vi "CODMn手动控制框.vi"(8 "Error in":errorcluster) -> ()   [LabVIEW 2016, in "斯坦道CODMn.lvlib"]
uses:
  <vilib>/Plasmionique/MB Master/MB Master.lvlib
panel:
  in  "氢氧化钠":bool
  in  "进样泵反转":bool
  in  "采水泵排":bool
  in  "采水泵进":bool
  in  "草酸钠":bool
  in  "高锰酸钾":bool
  in  "高锰酸钾滴定（10uL每滴）":bool
  in  "草酸钠泵排":bool
  in  "草酸钠泵进":bool
  in  "草酸钠泵复位":bool
  in  "高锰酸钾泵排":bool
  in  "高锰酸钾泵进":bool
  in  "高锰酸钾泵复位":bool
  in  "风扇":bool
  in  "排液":bool
  in  "搅拌":bool
  in  "加热":bool
  in  "硫酸":bool
  in  "加标回收样":bool
  in  "零点核查样":bool
  in  "标液":bool
  in  "纯水":bool
  in  "退出":bool
  in  "水样":bool
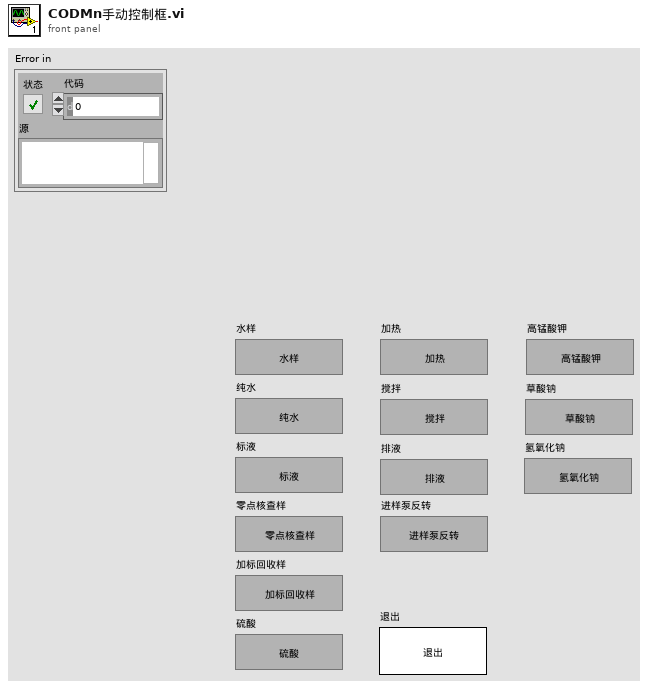
[diagram p1: front panel]
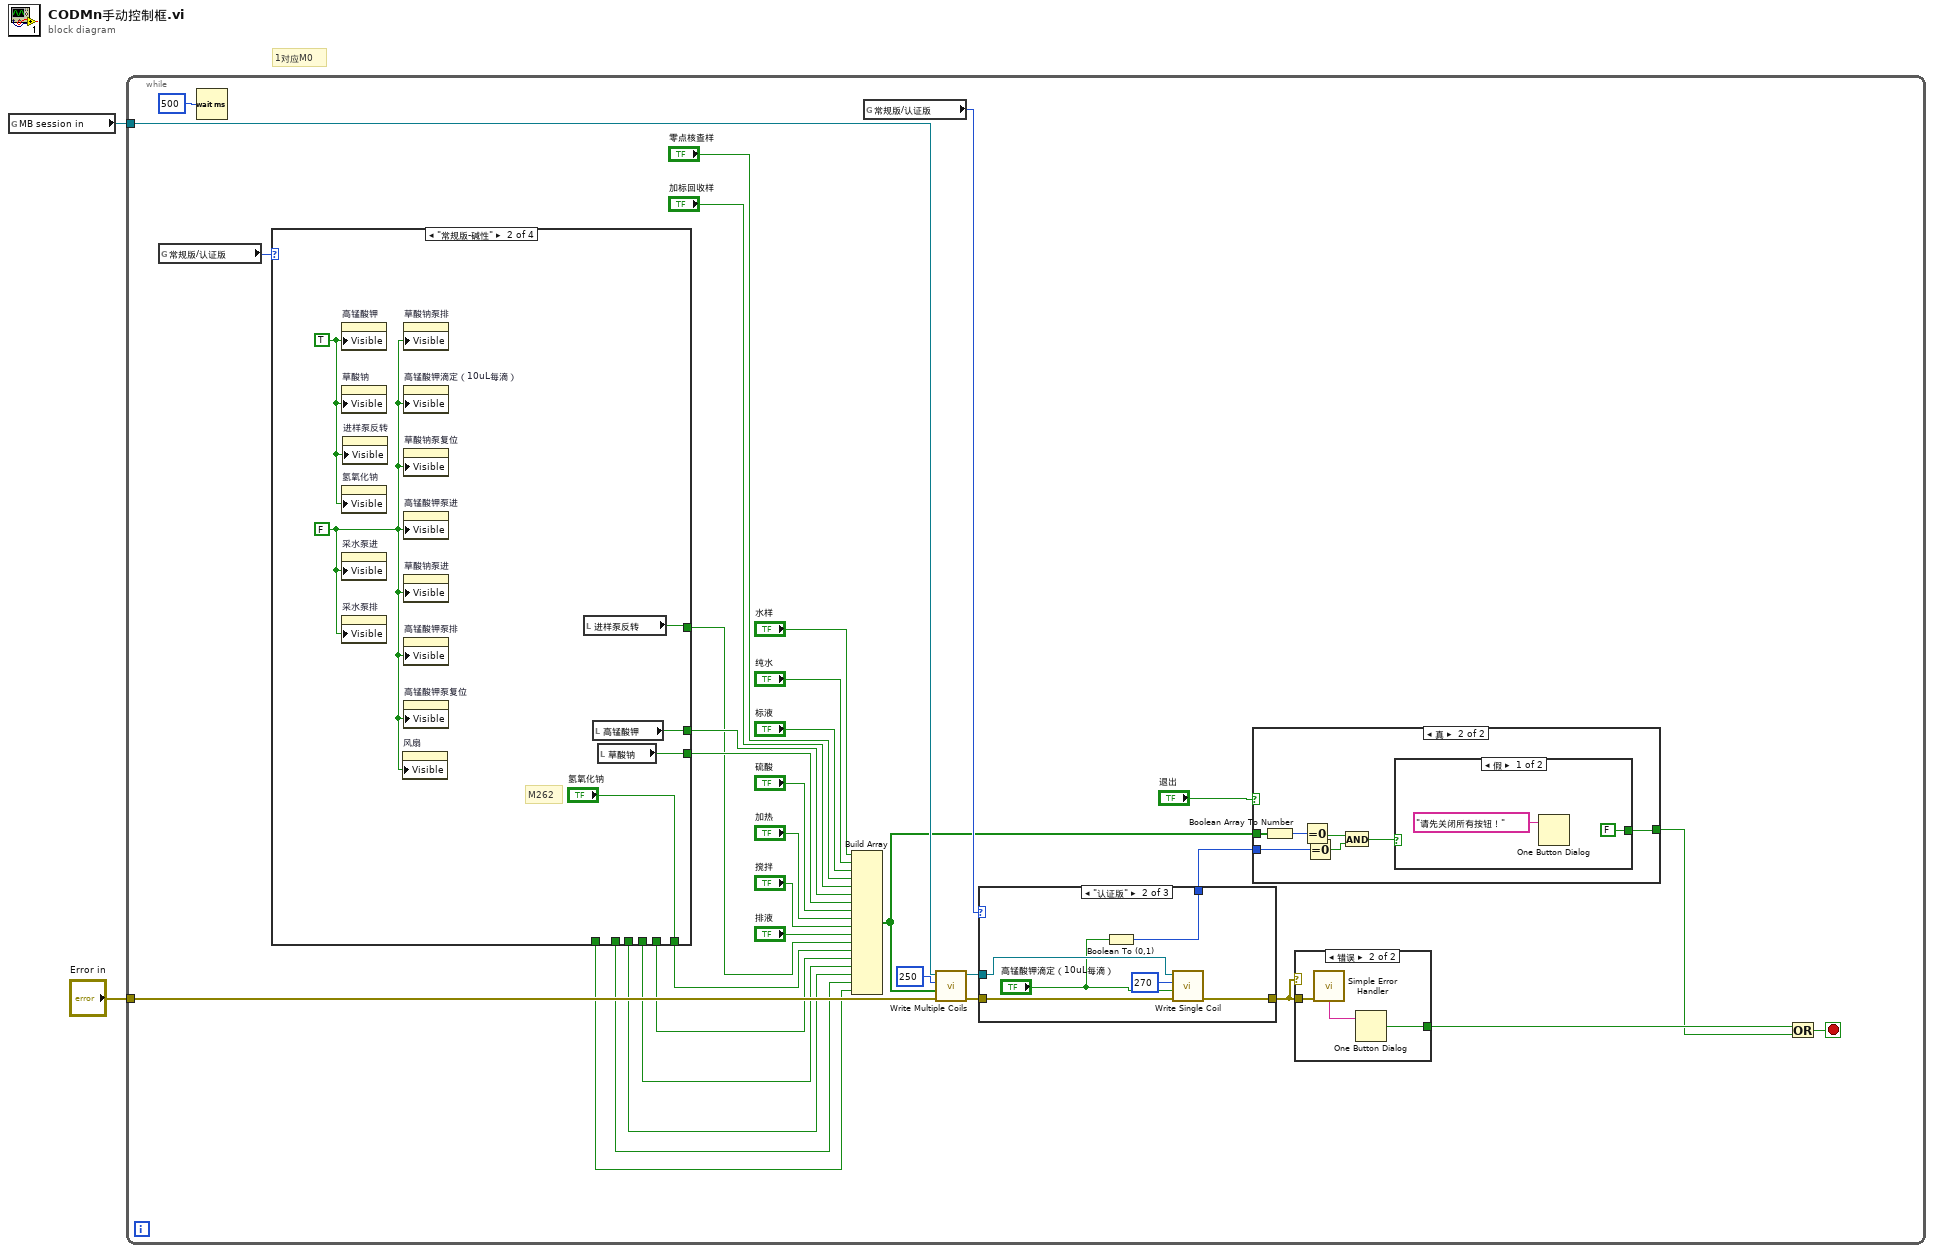
[diagram p0: block diagram]
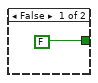
[diagram p2: hidden frame]
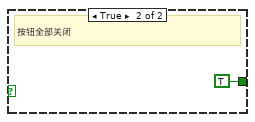
[diagram p3: hidden frame]
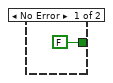
[diagram p4: hidden frame]
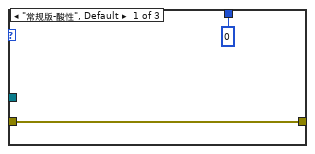
[diagram p5: hidden frame]
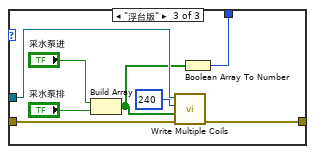
[diagram p6: hidden frame]
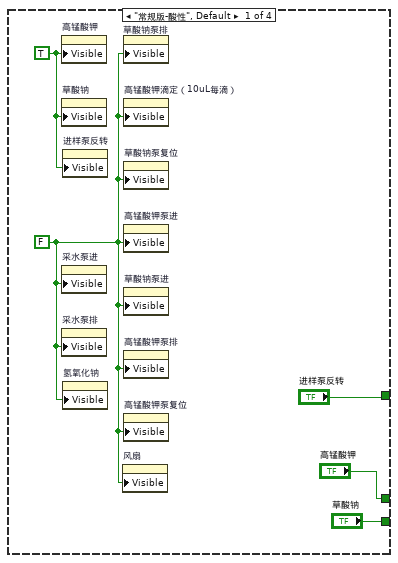
[diagram p7: hidden frame]
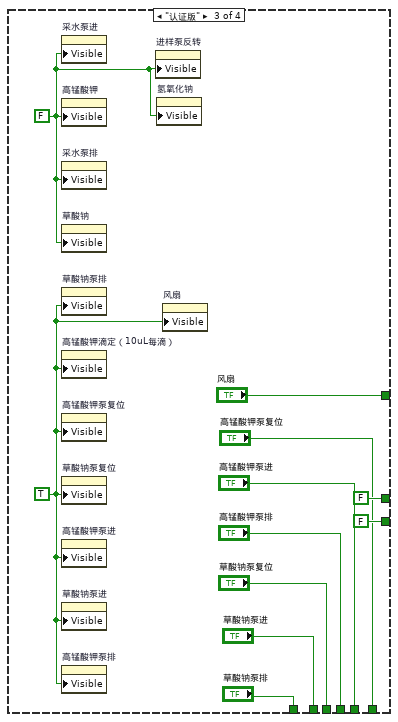
[diagram p8: hidden frame]
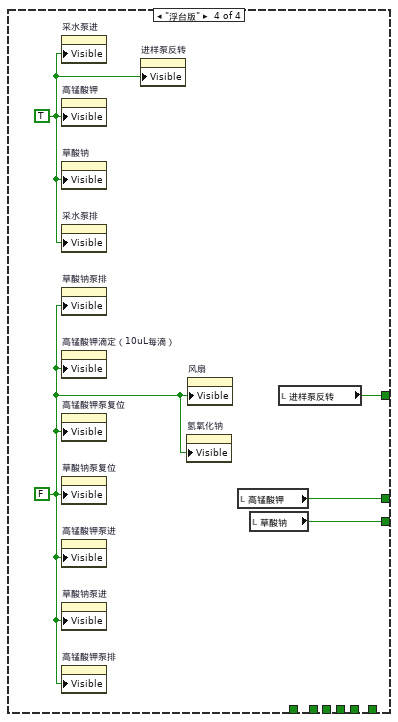
[diagram p9: hidden frame]
diagram:
  # "1对应M0"
  n1 = global read "COD浓度全局变量.vi" "MB session in"() -> (w1:refnum<class "MB_Master.lvclass">)
  n2 = while {
    tunnel: "Error in" -> [w24]
    tunnel: w1 -> [w19]
    stop <- w16 stop-if-true
    n3 = global read "CODMn断电保存全局变量.vi" "常规版/认证版"() -> (w15:enum16{"常规版-酸性", "常规版-碱性", "认证版", "浮台版"})
    n4 = Wait (ms)(milliseconds to wait=u32 500 ("等待时间（毫秒）")) -> ()  [unwired: 1 out]
    n5 = case shown="\"常规版-碱性\"" w15 {
      tunnel: ["高锰酸钾" w76 FALSE ("元素") w93] -> w21
      tunnel: ["草酸钠" w75 FALSE ("元素") w92] -> w20
      tunnel: [_ "氢氧化钠" "高锰酸钾泵复位" _] -> w13
      tunnel: [_ _ "高锰酸钾泵进" _] -> w12
      tunnel: [_ _ "高锰酸钾泵排" _] -> w11
      tunnel: [_ _ "草酸钠泵复位" _] -> w10
      tunnel: [_ _ "草酸钠泵进" _] -> w9
      tunnel: [_ _ "草酸钠泵排" _] -> w8
      tunnel: ["进样泵反转" w74 "风扇" w90] -> w7
      frame "常规版-酸性", Default {
        w67 = FALSE ("可见")
        w68 = TRUE ("可见")
        n6 = property on="高锰酸钾" class="Bool (严格)"("Visible"=w68) -> ()  [unwired: 2 in, 2 out]
        n7 = property on="草酸钠" class="Bool (严格)"("Visible"=w68) -> ()  [unwired: 2 in, 2 out]
        n8 = property on="采水泵进" class="Bool (严格)"("Visible"=w67) -> ()  [unwired: 2 in, 2 out]
        n9 = property on="采水泵排" class="Bool (严格)"("Visible"=w67) -> ()  [unwired: 2 in, 2 out]
        n10 = property on="进样泵反转" class="Bool (严格)"("Visible"=w68) -> ()  [unwired: 2 in, 2 out]
        n11 = property on="氢氧化钠" class="Bool (严格)"("Visible"=w67) -> ()  [unwired: 2 in, 2 out]
        n12 = property on="风扇" class="Bool (严格)"("Visible"=w67) -> ()  [unwired: 2 in, 2 out]
        n13 = property on="草酸钠泵排" class="Bool (严格)"("Visible"=w67) -> ()  [unwired: 2 in, 2 out]
        n14 = property on="高锰酸钾滴定（10uL每滴）" class="Bool (严格)"("Visible"=w67) -> ()  [unwired: 2 in, 2 out]
        n15 = property on="草酸钠泵复位" class="Bool (严格)"("Visible"=w67) -> ()  [unwired: 2 in, 2 out]
        n16 = property on="高锰酸钾泵进" class="Bool (严格)"("Visible"=w67) -> ()  [unwired: 2 in, 2 out]
        n17 = property on="草酸钠泵进" class="Bool (严格)"("Visible"=w67) -> ()  [unwired: 2 in, 2 out]
        n18 = property on="高锰酸钾泵排" class="Bool (严格)"("Visible"=w67) -> ()  [unwired: 2 in, 2 out]
        n19 = property on="高锰酸钾泵复位" class="Bool (严格)"("Visible"=w67) -> ()  [unwired: 2 in, 2 out]
      }
      frame "常规版-碱性" {
        w77 = FALSE ("可见")
        w72 = TRUE ("可见")
        # "M262"
        n20 = property on="高锰酸钾" class="Bool (严格)"("Visible"=w72) -> ()  [unwired: 2 in, 2 out]
        n21 = property on="草酸钠" class="Bool (严格)"("Visible"=w72) -> ()  [unwired: 2 in, 2 out]
        n22 = property on="氢氧化钠" class="Bool (严格)"("Visible"=w72) -> ()  [unwired: 2 in, 2 out]
        n23 = property on="采水泵进" class="Bool (严格)"("Visible"=w77) -> ()  [unwired: 2 in, 2 out]
        n24 = property on="采水泵排" class="Bool (严格)"("Visible"=w77) -> ()  [unwired: 2 in, 2 out]
        n25 = property on="进样泵反转" class="Bool (严格)"("Visible"=w72) -> ()  [unwired: 2 in, 2 out]
        n26 = property on="风扇" class="Bool (严格)"("Visible"=w77) -> ()  [unwired: 2 in, 2 out]
        n27 = property on="草酸钠泵排" class="Bool (严格)"("Visible"=w77) -> ()  [unwired: 2 in, 2 out]
        n28 = property on="高锰酸钾滴定（10uL每滴）" class="Bool (严格)"("Visible"=w77) -> ()  [unwired: 2 in, 2 out]
        n29 = property on="草酸钠泵复位" class="Bool (严格)"("Visible"=w77) -> ()  [unwired: 2 in, 2 out]
        n30 = property on="高锰酸钾泵进" class="Bool (严格)"("Visible"=w77) -> ()  [unwired: 2 in, 2 out]
        n31 = property on="草酸钠泵进" class="Bool (严格)"("Visible"=w77) -> ()  [unwired: 2 in, 2 out]
        n32 = property on="高锰酸钾泵排" class="Bool (严格)"("Visible"=w77) -> ()  [unwired: 2 in, 2 out]
        n33 = property on="高锰酸钾泵复位" class="Bool (严格)"("Visible"=w77) -> ()  [unwired: 2 in, 2 out]
        n34 = local read "进样泵反转"() -> (w74:bool)
        n35 = local read "高锰酸钾"() -> (w76:bool)
        n36 = local read "草酸钠"() -> (w75:bool)
      }
      frame "认证版" {
        w79 = TRUE ("可见")
        w78 = FALSE ("可见")
        n37 = property on="采水泵进" class="Bool (严格)"("Visible"=w78) -> ()  [unwired: 2 in, 2 out]
        n38 = property on="高锰酸钾" class="Bool (严格)"("Visible"=w78) -> ()  [unwired: 2 in, 2 out]
        n39 = property on="采水泵排" class="Bool (严格)"("Visible"=w78) -> ()  [unwired: 2 in, 2 out]
        n40 = property on="草酸钠" class="Bool (严格)"("Visible"=w78) -> ()  [unwired: 2 in, 2 out]
        n41 = property on="草酸钠泵排" class="Bool (严格)"("Visible"=w79) -> ()  [unwired: 2 in, 2 out]
        n42 = property on="高锰酸钾滴定（10uL每滴）" class="Bool (严格)"("Visible"=w79) -> ()  [unwired: 2 in, 2 out]
        n43 = property on="高锰酸钾泵复位" class="Bool (严格)"("Visible"=w79) -> ()  [unwired: 2 in, 2 out]
        n44 = property on="草酸钠泵复位" class="Bool (严格)"("Visible"=w79) -> ()  [unwired: 2 in, 2 out]
        n45 = property on="高锰酸钾泵进" class="Bool (严格)"("Visible"=w79) -> ()  [unwired: 2 in, 2 out]
        n46 = property on="草酸钠泵进" class="Bool (严格)"("Visible"=w79) -> ()  [unwired: 2 in, 2 out]
        n47 = property on="高锰酸钾泵排" class="Bool (严格)"("Visible"=w79) -> ()  [unwired: 2 in, 2 out]
        n48 = property on="进样泵反转" class="Bool (严格)"("Visible"=w78) -> ()  [unwired: 2 in, 2 out]
        n49 = property on="氢氧化钠" class="Bool (严格)"("Visible"=w78) -> ()  [unwired: 2 in, 2 out]
        n50 = property on="风扇" class="Bool (严格)"("Visible"=w79) -> ()  [unwired: 2 in, 2 out]
      }
      frame "浮台版" {
        w89 = FALSE ("可见")
        w91 = TRUE ("可见")
        n51 = property on="采水泵进" class="Bool (严格)"("Visible"=w91) -> ()  [unwired: 2 in, 2 out]
        n52 = property on="高锰酸钾" class="Bool (严格)"("Visible"=w91) -> ()  [unwired: 2 in, 2 out]
        n53 = property on="草酸钠" class="Bool (严格)"("Visible"=w91) -> ()  [unwired: 2 in, 2 out]
        n54 = property on="采水泵排" class="Bool (严格)"("Visible"=w91) -> ()  [unwired: 2 in, 2 out]
        n55 = property on="草酸钠泵排" class="Bool (严格)"("Visible"=w89) -> ()  [unwired: 2 in, 2 out]
        n56 = property on="高锰酸钾滴定（10uL每滴）" class="Bool (严格)"("Visible"=w89) -> ()  [unwired: 2 in, 2 out]
        n57 = property on="高锰酸钾泵复位" class="Bool (严格)"("Visible"=w89) -> ()  [unwired: 2 in, 2 out]
        n58 = property on="草酸钠泵复位" class="Bool (严格)"("Visible"=w89) -> ()  [unwired: 2 in, 2 out]
        n59 = property on="高锰酸钾泵进" class="Bool (严格)"("Visible"=w89) -> ()  [unwired: 2 in, 2 out]
        n60 = property on="草酸钠泵进" class="Bool (严格)"("Visible"=w89) -> ()  [unwired: 2 in, 2 out]
        n61 = property on="高锰酸钾泵排" class="Bool (严格)"("Visible"=w89) -> ()  [unwired: 2 in, 2 out]
        n62 = property on="进样泵反转" class="Bool (严格)"("Visible"=w91) -> ()  [unwired: 2 in, 2 out]
        n63 = property on="氢氧化钠" class="Bool (严格)"("Visible"=w89) -> ()  [unwired: 2 in, 2 out]
        n64 = property on="风扇" class="Bool (严格)"("Visible"=w89) -> ()  [unwired: 2 in, 2 out]
        n65 = local read "高锰酸钾"() -> (w93:bool)
        n66 = local read "草酸钠"() -> (w92:bool)
        n67 = local read "进样泵反转"() -> (w90:bool)
      }
    }
    n68 = Build Array("水样", "纯水", "标液", "零点核查样", "加标回收样", w21, w20, "硫酸", "加热", "搅拌", "排液", w7, w13, w12, w11, w10, w9, w8) -> (w6:bool[])
    n69 = global read "CODMn断电保存全局变量.vi" "常规版/认证版"() -> (w14:enum16{"常规版-酸性", "常规版-碱性", "认证版", "浮台版"})
    n70 = call <vilib>:"Write Multiple Coils.vi"("error in (no error)"=w24, "values"=w6, "starting address"=u16 250, "MB session in"=w19) -> ("error out"=w22:errorcluster, "MB session out"=w23:refnum<class "MB_Master.lvclass">)  [unwired: 6 in]
    n71 = case shown="\"认证版\"" w14 {
      tunnel: w23 -> [_ w58 w66]
      tunnel: w22 -> [w52 w57 w65]
      tunnel: [w52 w55 w61] -> w18
      tunnel: [u32 0 w53 w59] -> w5
      frame "常规版-酸性", Default {
      }
      frame "认证版" {
        n72 = Boolean To (0,1)(Boolean="高锰酸钾滴定（10uL每滴）") -> (0, 1=w53:i16)
        n73 = call <vilib>:"Write Single Coil.vi"("error in (no error)"=w57, "value"="高锰酸钾滴定（10uL每滴）", "address"=u16 270 ("starting address"), "MB session in"=w58) -> ("error out"=w55:errorcluster)  [unwired: 6 in, 1 out]
      }
      frame "浮台版" {
        n74 = Build Array("采水泵进", "采水泵排") -> (w60:bool[])
        n75 = call <vilib>:"Write Multiple Coils.vi"("error in (no error)"=w65, "values"=w60, "starting address"=u16 240, "MB session in"=w66) -> ("error out"=w61:errorcluster)  [unwired: 6 in, 1 out]
        n76 = Boolean Array To Number(Boolean array=w60) -> (number=w59:u32)
      }
    }
    n77 = case shown="真" "退出" {
      tunnel: w6 -> [_ w43]
      tunnel: w5 -> [_ w41]
      tunnel: [FALSE w37] -> w3
      frame False {
      }
      frame True {
        n78 = Boolean Array To Number(Boolean array=w43) -> (number=w42:u32)
        n79 = Equal To 0?(x=w42) -> (x = 0?=w40:bool)
        n80 = Equal To 0?(x=w41) -> (x = 0?=w39:bool)
        n81 = And(x=w40, y=w39) -> (x .and. y?=w38:bool)
        n82 = case shown="假" w38 {
          tunnel: [FALSE TRUE] -> w37
          frame False {
            n83 = One Button Dialog(message="请先关闭所有按钮！" ("消息")) -> ()  [unwired: 1 in, 1 out]
          }
          frame True {
            # "按钮全部关闭"
          }
        }
      }
    }
    n84 = case shown="错误" w18 {
      tunnel: w18 -> [_ w50]
      tunnel: [FALSE ("true") w48] -> w17
      frame No Error {
      }
      frame Error {
        n85 = call <vilib>:"Simple Error Handler.vi"("error in (no error)"=w50) -> ("message"=w49:string)  [unwired: 4 in, 4 out]
        n86 = One Button Dialog(message=w49) -> (true=w48:bool)  [unwired: 1 in]
      }
    }
    n87 = Or(x=w17, y=w3) -> (x .or. y?=w16:bool)
  }
